vi "Remove Module.vi"(8 "error in":errorcluster, 10 "module path":string, 11 "routing and faulting in":T1 format="%.0x") -> (0 "error out":errorcluster, 3 "routing and faulting out":T1 format="%.0x")   [LabVIEW 2020, in "Routing and Faulting Scripting.lvlib"]
uses:
  Routing and Faulting Scripting.lvlib
  <vilib>/NI VeriStand/Custom Device API/Custom Device Item Ref.ctl
  NationalInstruments.VeriStand.SystemStorage
  Constants/Scripting Constants.vi
  <vilib>/NI VeriStand/Custom Device API/Custom Device API.lvlib
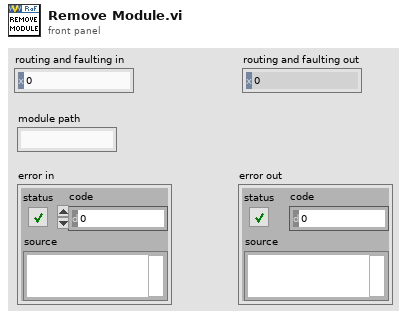
[diagram p1: front panel]
types:
  T1 = typedef "Custom Device API.lvlib/Custom Device Item Ref.ctl" = u64
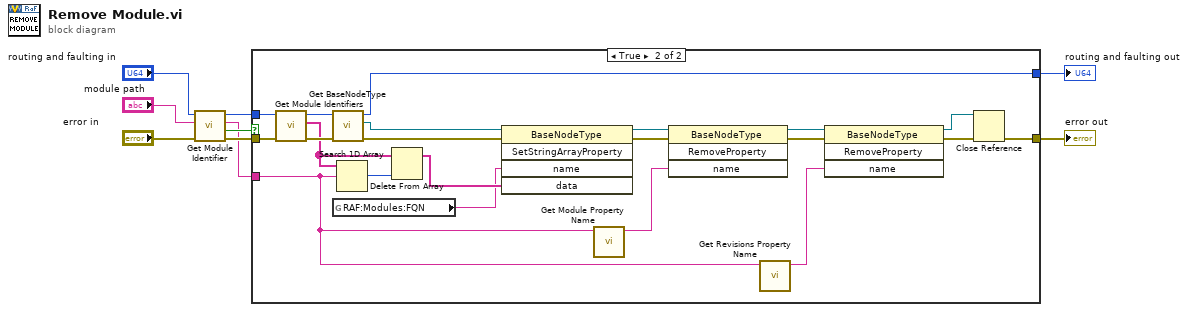
[diagram p0: block diagram]
diagram:
  n1 = call "Get Module Identifier.vi"("error in"="error in", "module path"="module path", "routing and faulting in"="routing and faulting in") -> ("error out"=w7:errorcluster, "found?"=w6:bool, "module identifier"=w4:string, "routing and faulting out"=w5:T1)  [unwired: 5 in]
  n2 = case shown="True" w6 {
    tunnel: w7 -> [w11 w30]
    tunnel: w5 -> [w10 w29]
    tunnel: w4 -> [_ w12]
    tunnel: [w11 w32] -> w3
    tunnel: [w10 w18] -> w1
    frame False {
    }
    frame True {
      n3 = call "Get Module Identifiers.vi"("error in"=w30, "routing and faulting in"=w29) -> ("error out"=w28:errorcluster, "module Identifier"=w26:string[], "routing and faulting out"=w27:T1)  [unwired: 7 in]
      n4 = call "Get BaseNodeType.vi"("error in"=w28, "item in"=w27) -> ("error out"=w24:errorcluster, "BaseNodeType"=w23:refnum<k24>, "item out"=w18:T1)  [unwired: 7 in]
      n5 = global read "Scripting Constants.vi" "RAF:Modules:FQN"() -> (w21:string)
      n6 = Search 1D Array(1D array=w26, element=w12) -> (index of element=w25:i32)  [unwired: 1 in]
      n7 = Delete From Array(array=w26, index=w25) -> (array with subset deleted=w22:string[])  [unwired: 1 in, 1 out]
      n8 = invoke class="BaseNodeType" method="SetStringArrayProperty"(reference=w23, error in=w24, "name"=w21, "data"=w22) -> (reference out=w19:refnum<k24>, error out=w20:errorcluster)  [unwired: 1 in, 3 out]
      n9 = call "Get Module Property Name.vi"("module identifier"=w12) -> ("module property name"=w31:string)  [unwired: 10 in]
      n10 = invoke class="BaseNodeType" method="RemoveProperty"(reference=w19, error in=w20, "name"=w31) -> (reference out=w14:refnum<k24>, error out=w15:errorcluster)  [unwired: 1 in, 2 out]
      n11 = call "Get Revisions Property Name.vi"("module identifier"=w12) -> ("module revision property name"=w13:string)  [unwired: 10 in]
      n12 = invoke class="BaseNodeType" method="RemoveProperty"(reference=w14, error in=w15, "name"=w13) -> (reference out=w16:refnum<k24>, error out=w17:errorcluster)  [unwired: 1 in, 2 out]
      n13 = Close Reference(reference=w16, error in (no error)=w17) -> (error out=w32:errorcluster)
    }
  }
  "error out" <- w3
  "routing and faulting out" <- w1
